vi "5.0 EMGtoOMG LIVE.vi"() -> ()   [LabVIEW 2018]
uses:
  <vilib>/express/express analysis/Spectral/Block/exnSpectralBlock spectral measurements power poly.vi
  <vilib>/express/express analysis/Spectral/Block/exnSpectralBlock spectral measurements power DDT.vi
  <vilib>/express/express analysis/Spectral/XNode/ExpressSpectralMeasurementsBlockNode.xnode
panel:
  out "?":bool
  out "?":bool
  out "?":bool
  out "?":bool
  out "?":bool
  out "?":bool
  out "?":bool
  out "?":bool
  out "?":bool
  in  "file path (use dialog) 2":path
  in  "Numeric 3":dbl=0.05 format="%#_13g"
  in  "Numeric 2":dbl=0.05 format="%#_13g"
  in  "Numeric":dbl=0.05 format="%#_13g"
  in  "rate":dbl=5000.0
  in  "sample size":i32=5000
  out "RMS 3":dbl
  out "RMS 2":dbl
  out "RMS":dbl
  out "return value":string
  out "charSearch":dbl[](array[numeric])
  out "setID":dbl[](array[numeric])
  in  "stop":bool
  in  "module path":path
  # "1-1-3     3 (x8) \"G\"     1-2-1     3 (x4) \"o\"     2\n\n1-1-2     3 (x2) \"b\"     1-2-1     3 (x1) \"l\"     1-2-2     3 (x5) \"u\"     1-1-2     3 (x5) \"e\"     2\n\n1-3-1     3 (x4) \"!\"     1-1-1     2     3 (x2)     2     1"
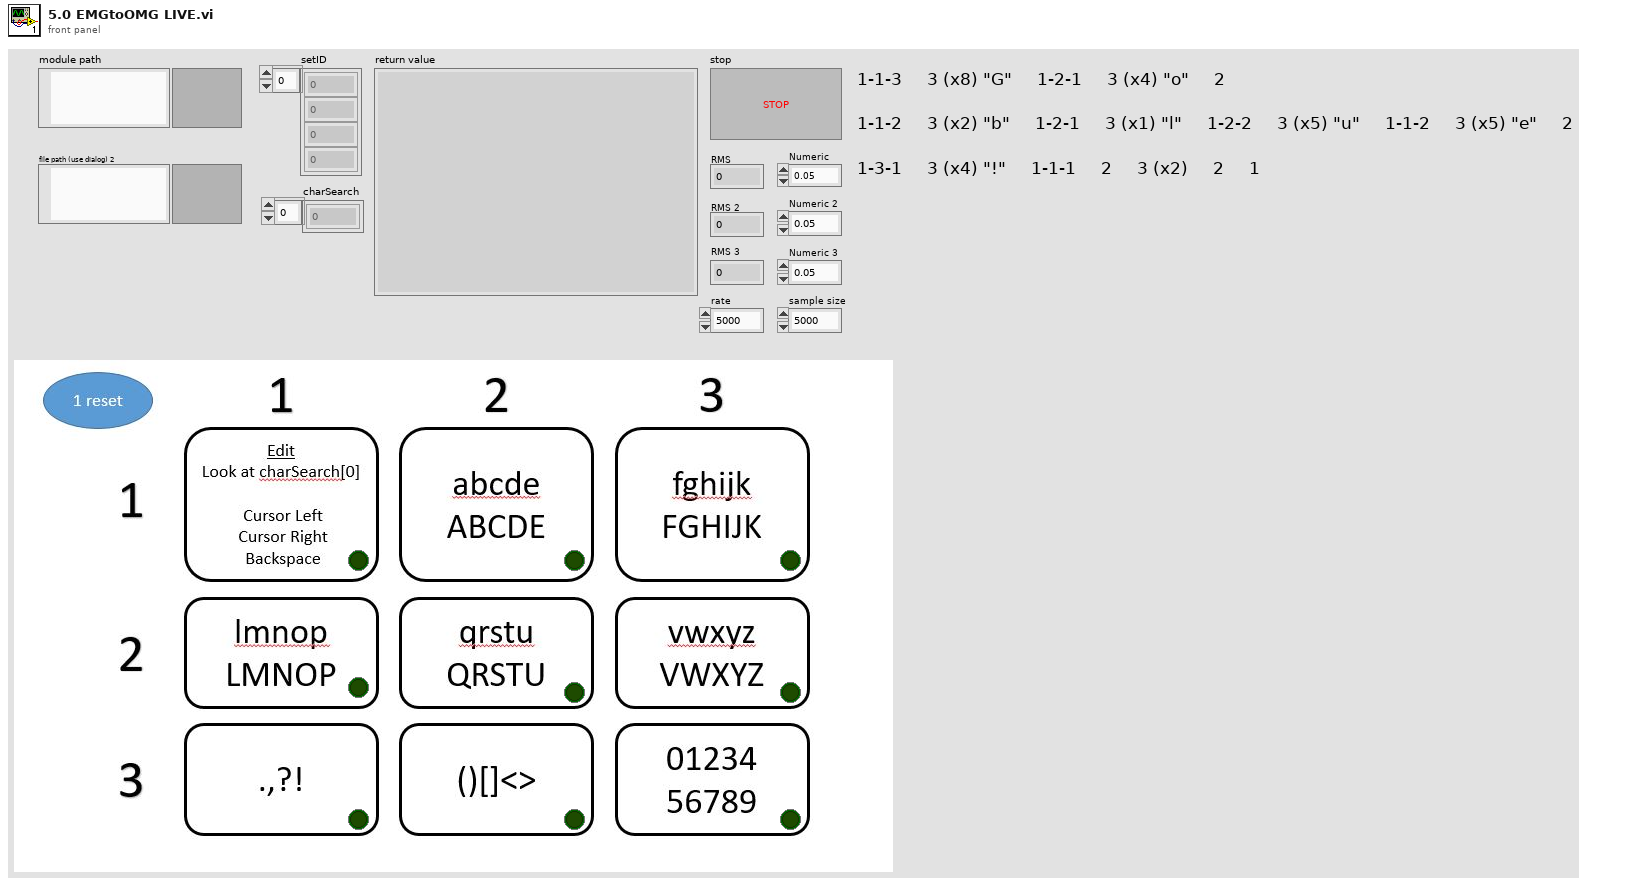
[diagram p1: front panel]
types:
  T1 = enum16{"open", "replace", "create", "open or create", "replace or create", "replace or create with confirmation"}
  T2 = cluster{"averaging mode":u16, "weighting mode":u16, "number of averages":u32}
  T3 = cluster{"dB On (F)":bool, "unwrap phase (F)":bool, "convert to degree (F)":bool}
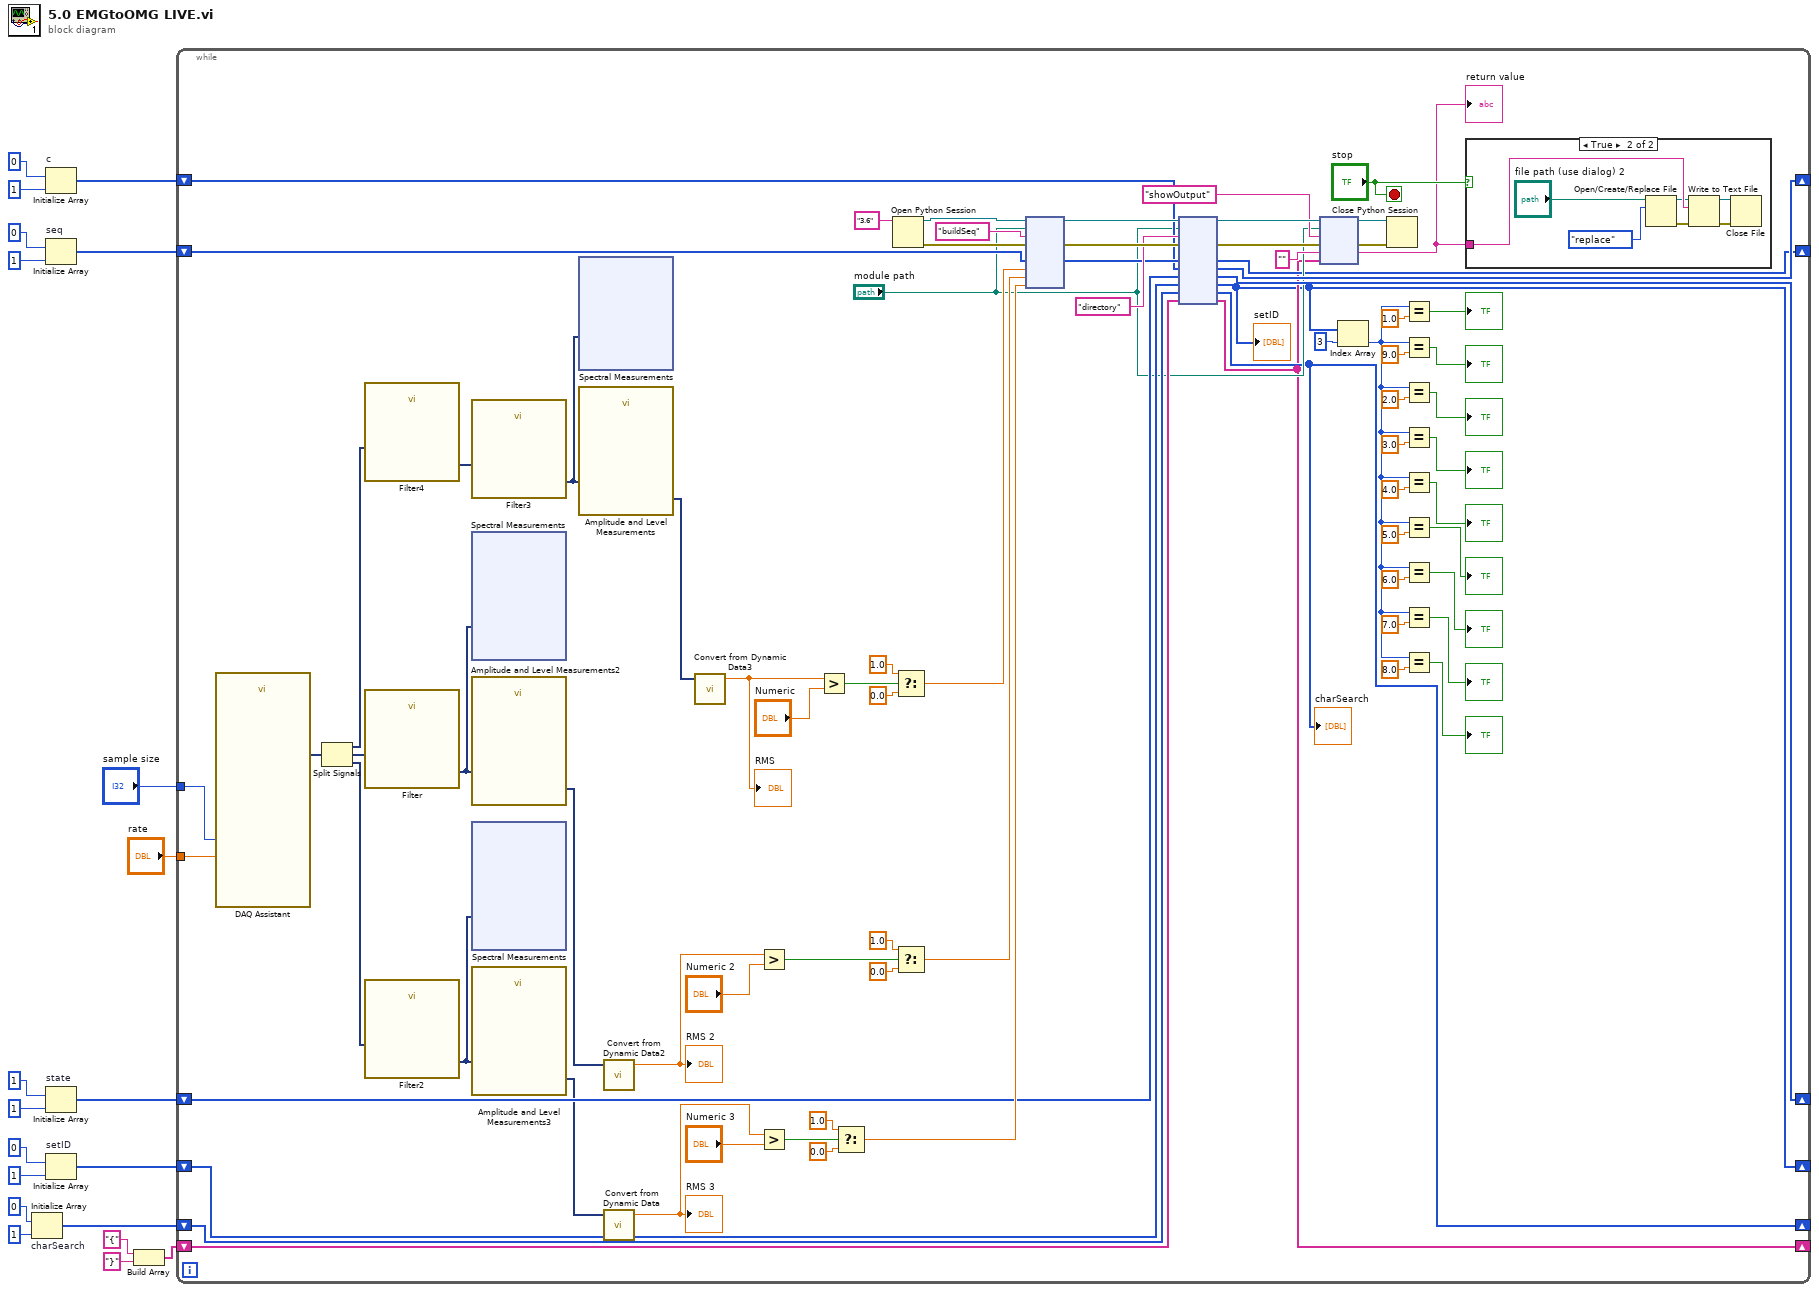
[diagram p0: block diagram]
diagram:
  n1 = Initialize Array "charSearch"(0, 1 ("dimension size")) -> (w15:i32[])
  n2 = Initialize Array "c"(0, 1 ("dimension size")) -> (w13:i32[])
  n3 = Initialize Array "seq"(0, 1 ("dimension size")) -> (w20:i32[])
  n4 = Initialize Array "state"(1, 1 ("dimension size")) -> (w10:i32[])
  n5 = Initialize Array "setID"(0, 1 ("dimension size")) -> (w16:i32[])
  n6 = Build Array("{", "}") -> (w7:string[])
  n7 = while {
    shift-right: [w43] -> _
    shift-left: w20 -> [w93]
    shift-right: [w41] -> _
    shift-left: w16 -> [w82]
    shift-right: [w68] -> _
    shift-left: w15 -> [w81]
    shift-right: [w42] -> _
    shift-left: w7 -> [w80]
    shift-right: [w78] -> _
    shift-left: w10 -> [w79]
    shift-right: [w76] -> _
    shift-left: w13 -> [w77]
    tunnel: "sample size" -> [w47]
    tunnel: "rate" -> [w46]
    stop <- "stop" stop-if-true
    n8 = call "DAQ Assistant"("rate"=w46, "number of samples"=w47) -> ("data"=w65:dynamicdata)  [unwired: 15 in, 2 out]
    n9 = Split Signals(w65) -> (w61:dynamicdata, w64:dynamicdata, w63:dynamicdata)  [unwired: 3 in]
    n10 = call "Filter4"("Signal"=w61) -> ("Filtered Signal"=w60:dynamicdata)  [unwired: 9 in, 1 out]
    n11 = call "Filter"("Signal"=w64) -> ("Filtered Signal"=w67:dynamicdata)  [unwired: 9 in, 1 out]
    n12 = call "Filter2"("Signal"=w63) -> ("Filtered Signal"=w66:dynamicdata)  [unwired: 9 in, 1 out]
    n13 = call "Filter3"("Signal"=w60) -> ("Filtered Signal"=w62:dynamicdata)  [unwired: 9 in, 1 out]
    n14 = xnode "Spectral Measurements"("Signals"=w67) -> ()  [unwired: 1 in, 2 out]
    n15 = call "Amplitude and Level Measurements2"("Signals"=w67) -> ("RMS"=w57:dynamicdata)  [unwired: 13 in, 1 out]
    n16 = xnode "Spectral Measurements"("Signals"=w66) -> ()  [unwired: 1 in, 2 out]
    n17 = call "Amplitude and Level Measurements3"("Signals"=w66) -> ("RMS"=w59:dynamicdata)  [unwired: 13 in, 1 out]
    n18 = xnode "Spectral Measurements"("Signals"=w62) -> ()  [unwired: 1 in, 2 out]
    n19 = call "Amplitude and Level Measurements"("Signals"=w62) -> ("RMS"=w55:dynamicdata)  [unwired: 13 in, 1 out]
    n20 = call "Convert from Dynamic Data2"("Dynamic Data Type"=w57) -> ("Scalar"=w51:dbl)  [unwired: 3 in]
    "RMS 2" <- w51
    n21 = call "Convert from Dynamic Data"("Dynamic Data Type"=w59) -> ("Scalar"=w53:dbl)  [unwired: 3 in]
    "RMS 3" <- w53
    n22 = call "Convert from Dynamic Data3"("Dynamic Data Type"=w55) -> ("Scalar"=w50:dbl)  [unwired: 3 in]
    "RMS" <- w50
    n23 = Greater?(x=w51, y="Numeric 2") -> (0:w49:bool)
    n24 = Greater?(x=w53, y="Numeric 3") -> (0:w52:bool)
    n25 = Greater?(x=w50, y="Numeric") -> (0:w48:bool)
    n26 = Select(t=1.0, s=w52, f=0.0) -> (s? t:f=w87:dbl)
    n27 = Open Python Session(python version="3.6" ("Python version")) -> (session out=w99:refnum<k35>, error out=w98:errorcluster)  [unwired: 2 in]
    n28 = Select(t=1.0, s=w48, f=0.0) -> (s? t:f=w96:dbl)
    n29 = Select(t=1.0, s=w49, f=0.0) -> (s? t:f=w88:dbl)
    n30 = node(w99, "module path", "buildSeq" ("function name"), w98, w93, w96, w88, w87) -> (w86:refnum<k35>, w85:errorcluster, w83:i32[])  [unwired: 5 in, 2 out]
    n31 = node(w86, "module path", "directory" ("function name"), w85, w83, w77, w79, w82, w81, w80) -> (w74:refnum<k35>, w72:errorcluster, w43:i32[], w76:i32[], w78:i32[], w41:i32[], w68:i32[], w42:string[])  [unwired: 2 in, 2 out]
    "setID" <- w41
    "charSearch" <- w68
    n32 = node(w74, "module path", "showOutput" ("function name"), w72, "", w42) -> (w73:refnum<k35>, w71:errorcluster, w44:string)  [unwired: 1 in, 2 out]
    "return value" <- w44
    n33 = Index Array(array=w41, index=3) -> (element=w21:i32)
    n34 = Close Python Session(session in=w73, error in=w71) -> ()  [unwired: 1 out]
    n35 = Equal?(x=w21, y=1.0) -> (x = y?=→"?":bool)
    n36 = Equal?(x=w21, y=9.0) -> (x = y?=→"?":bool)
    n37 = Equal?(x=w21, y=2.0) -> (x = y?=→"?":bool)
    n38 = Equal?(x=w21, y=3.0) -> (x = y?=→"?":bool)
    n39 = Equal?(x=w21, y=4.0) -> (x = y?=→"?":bool)
    n40 = Equal?(x=w21, y=5.0) -> (x = y?=→"?":bool)
    n41 = Equal?(x=w21, y=6.0) -> (x = y?=→"?":bool)
    n42 = Equal?(x=w21, y=7.0) -> (x = y?=→"?":bool)
    n43 = Equal?(x=w21, y=8.0) -> (x = y?=→"?":bool)
    n44 = case shown="True" "stop" {
      tunnel: w44 -> [_ w107]
      frame False {
      }
      frame True {
        n45 = Open/Create/Replace File(file path (use dialog)="file path (use dialog) 2", operation (0:open)=T1."replace") -> (refnum out=w103:refnum<file>, error out=w104:errorcluster)  [unwired: 4 in, 1 out]
        n46 = Write to Text File(file (use dialog)=w103, text=w107, error in=w104) -> (refnum out=w105:refnum<file>, error out=w106:errorcluster)  [unwired: 1 in, 1 out]
        n47 = Close File(refnum=w105, error in=w106) -> ()  [unwired: 2 out]
      }
    }
  }
